vi "FL_Make_Track_overlay.vi"(4 "Pen properties":T1, 5 "Full track array":T2(array[cluster]), 6 "Colors array input":u32[](array[colorbox]), 7 "Picture in":picture) -> (1 "Picture out":picture)   [LabVIEW 2016]
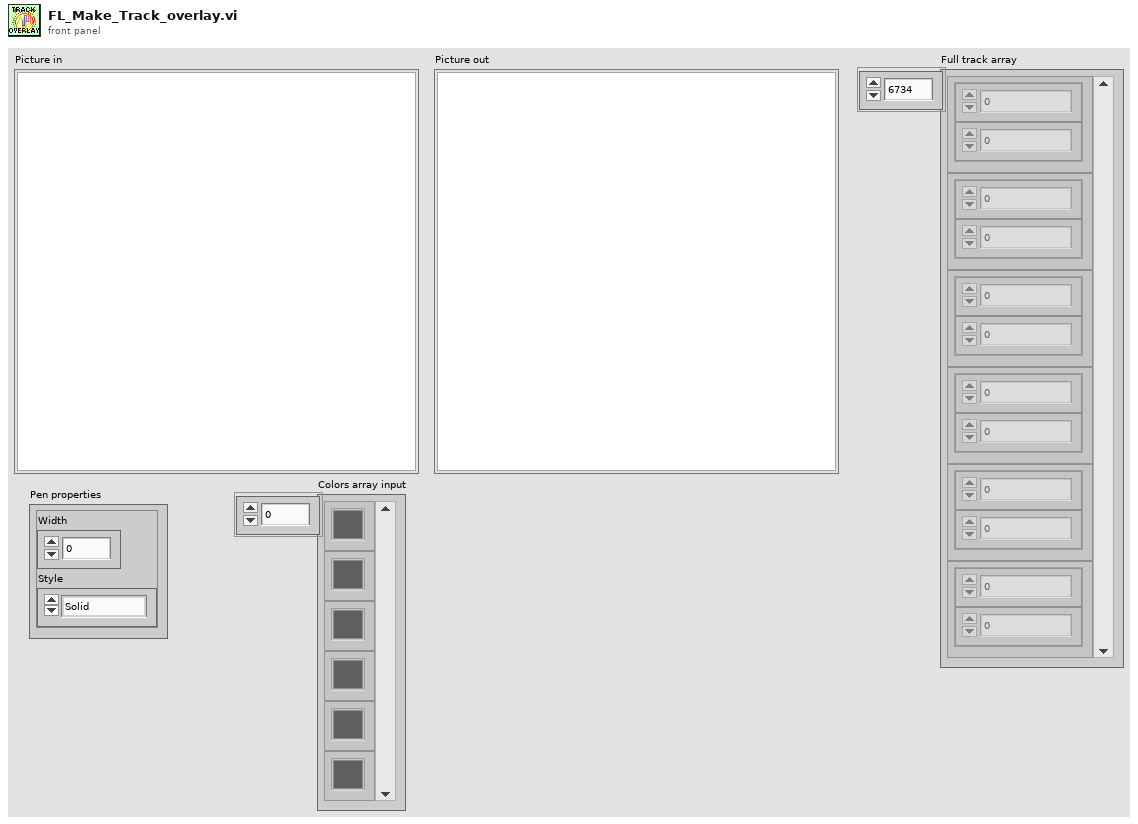
[diagram p1: front panel]
types:
  T1 = cluster{"Width":u16, "Style":enum32{"Solid", "Dash", "Dot", "DashDot", "DashDotDot"}}
  T2 = cluster{"Numeric Control":dbl, "Numeric Control":dbl}[]
  T3 = cluster{"Numeric Control":dbl, "Numeric Control":dbl}
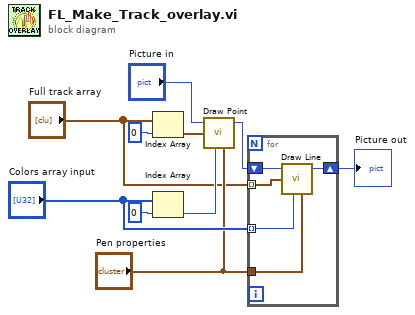
[diagram p0: block diagram]
diagram:
  n1 = Index Array(array="Full track array", index=0) -> (element=w2:T3)
  n2 = Index Array(array="Colors array input", index=0) -> (element=w5:u32)
  n3 = call <vilib>:"Draw Point.vi"("picture"="Picture in", "point(x,y)"=w2, "color(black)"=w5, "pen"="Pen properties") -> ("new picture"=w9:picture)  [unwired: 5 in]
  n4 = for {
    tunnel: "Pen properties" -> [w15]
    shift-right: [w14] -> w1
    shift-left: w9 -> [w12]
    tunnel: "Full track array" -> [w13] mode=indexing
    tunnel: "Colors array input" -> [w11] mode=indexing
    n5 = call <vilib>:"Draw Line.vi"("picture"=w12, "end point"=w13, "color(black)"=w11, "pen"=w15) -> ("new picture"=w14:picture)  [unwired: 5 in]
  }
  "Picture out" <- w1
